vi "resultsColumnsFilename.vi"(10 "chValuesIn":string[](array[string]), 11 "chNamesIn":string[](array[string])) -> (2 "chValuesOut":string[](array[string]), 3 "chNamesOut":string[](array[string]))   [LabVIEW 2020]
uses:
  Globals/Meas_global.vi
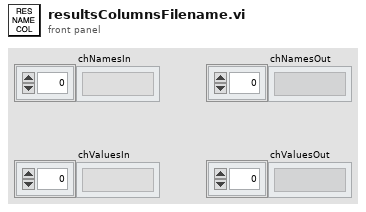
[diagram p1: front panel]
types:
  T1 = typedef "Post_Process.ctl" = enum16{"Take New Data", "Post Process Raw Data File"}
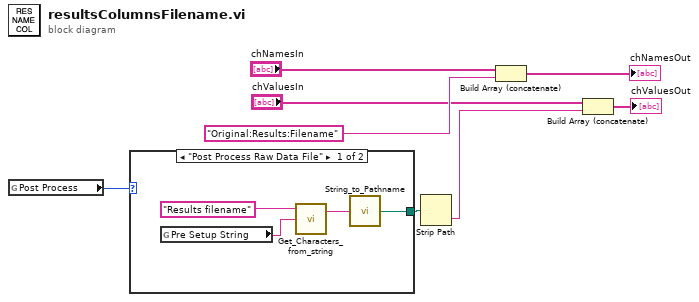
[diagram p0: block diagram]
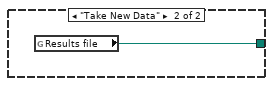
[diagram p2: hidden frame]
diagram:
  n1 = global read "Meas_global.vi" "Post Process"() -> (w8:T1)
  n2 = case shown="\"Post Process Raw Data File\"" w8 {
    tunnel: [w9 w13] -> w2
    frame "Post Process Raw Data File" {
      n3 = global read "Meas_global.vi" "Pre Setup String"() -> (w12:string)
      n4 = call "Get_Characters_from_string.vi"("Input string"=w12, "Variable name"="Results filename") -> ("Value"=w10:string)  [unwired: 1 in, 1 out]
      n5 = call "String_to_Pathname.vi"("Input String"=w10) -> ("path"=w9:path)
    }
    frame "Take New Data" {
      n6 = global read "Meas_global.vi" "Results file"() -> (w13:path)
    }
  }
  n7 = Strip Path(path=w2) -> (name=w3:string)  [unwired: 1 out]
  n8 = Build Array (concatenate)("chNamesIn", "Original:Results:Filename") -> (→"chNamesOut":string[])
  n9 = Build Array (concatenate)("chValuesIn", w3) -> (→"chValuesOut":string[])
